vi "Default Role.vi"(11 "Roles API in":refnum<class "Roles API.lvclass">) -> (2 "Default Role":string, 3 "Roles API out":refnum<class "Roles API.lvclass">)   [LabVIEW 2020, in "Volatus.lvlib" / "Roles API.lvclass"]
uses:
  Roles API.lvclass
  Roles API.lvclass/Roles API.ctl
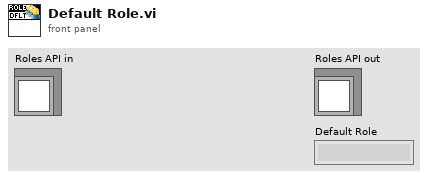
[diagram p1: front panel]
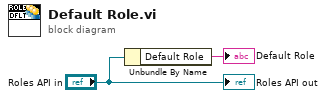
[diagram p0: block diagram]
diagram:
  n1 = Unbundle By Name("Roles API in") -> ("Default Role"=→"Default Role":string)
  "Roles API out" <- "Roles API in"
